vi "tbhwithreinitialize.vi"(1 "Gain":dbl=0.001, 2 "Act":dbl, 3 "Cmd":dbl) -> (0 "Out":dbl)   [LabVIEW 2016]
panel:
  out "Error":dbl=-485.8692080184028
  out "H0":dbl=-30.366825501150174
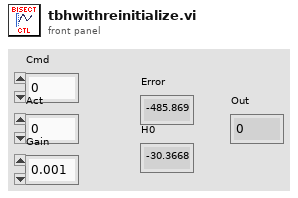
[diagram p1: front panel]
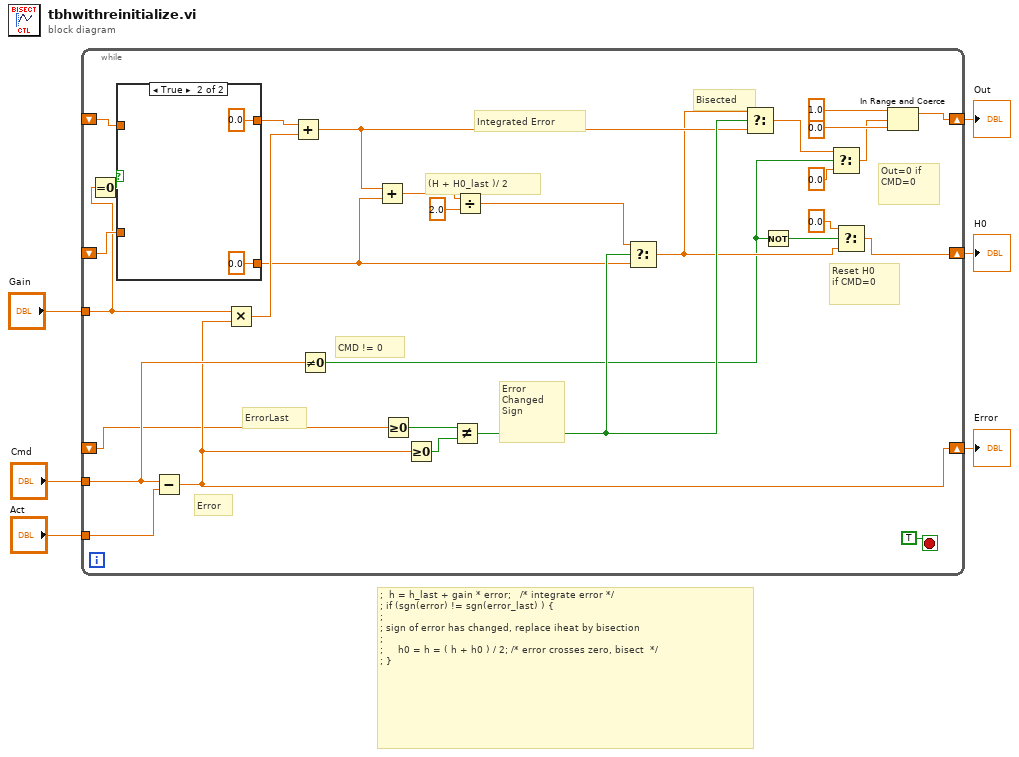
[diagram p0: block diagram]
diagram:
  # "; \th = h_last + gain * error;\t\t\t/* integrate error */\n;\tif (sgn(error) != sgn(error_last) ) {\n;\n; sign of error has changed, replace iheat by bisection\n;\n;\t    h0 = h = ( h + h0 ) / 2;\t/* error crosses zero, bisect  */\n;\t}"
  n1 = while {
    shift-right: [w20] -> w2
    shift-left: _ -> [w10]
    tunnel: "Cmd" -> [w22]
    tunnel: "Act" -> [w35]
    shift-right: [w15] -> w1
    shift-left: _ -> [w14]
    shift-right: [w26] -> w3
    shift-left: _ -> [w12]
    tunnel: "Gain" -> [w8]
    stop <- TRUE stop-if-true
    # "CMD != 0"
    # "Out=0 if\nCMD=0"
    # "Reset H0\nif CMD=0"
    # "ErrorLast"
    # "Bisected"
    # "Integrated Error"
    # "(H + H0_last )/ 2"
    # "Error\nChanged\nSign"
    # "Error"
    n2 = Equal To 0?(x=w8) -> (x = 0?=w7:bool)
    n3 = case shown="True" w7 {
      tunnel: w12 -> [w37 _]
      tunnel: [w37 0.0 ("upper limit")] -> w11
      tunnel: w10 -> [w38 _]
      tunnel: [w38 0.0 ("t")] -> w9
      frame False {
      }
      frame True {
      }
    }
    n4 = Subtract(x=w22, y=w35) -> (x-y=w15:dbl)
    n5 = Multiply(x=w8, y=w15) -> (x*y=w33:dbl)
    n6 = Add(x=w11, y=w33) -> (x+y=w32:dbl)
    n7 = Not Equal To 0?(x=w22) -> (x != 0?=w19:bool)
    n8 = Add(x=w32, y=w9) -> (x+y=w31:dbl)
    n9 = Greater Or Equal To 0?(x=w14) -> (x >= 0?=w13:bool)
    n10 = Greater Or Equal To 0?(x=w15) -> (x >= 0?=w16:bool)
    n11 = Not Equal?(x=w13, y=w16) -> (x != y?=w34:bool)
    n12 = Divide(x=w31, y=2.0) -> (x/y=w29:dbl)
    n13 = Select(t=w29, s=w34, f=w9) -> (s? t:f=w21:dbl)
    n14 = Select(t=w21, s=w34, f=w32) -> (s? t:f=w25:dbl)
    n15 = Not(x=w19) -> (.not. x?=w18:bool)
    n16 = Select(t=w25, s=w19, f=0.0) -> (s? t:f=w24:dbl)
    n17 = Select(t=0.0, s=w18, f=w21) -> (s? t:f=w20:dbl)
    n18 = In Range and Coerce(upper limit=1.0, x=w24, lower limit=0.0) -> (coerced(x)=w26:dbl)  [unwired: 1 out]
  }
  "Out" <- w3
  "H0" <- w2
  "Error" <- w1
